vi "Laser349_RS232_Write_settings.vi"(7 "Command Status":T1, 8 "error in (no error)":errorcluster, 10 "Input value":dbl, 11 "Laser349 in":refnum<class "Laser349.lvclass">) -> (0 "error out":errorcluster, 3 "Laser349 out":refnum<class "Laser349.lvclass">)   [LabVIEW 2018, in "Laser349.lvclass"]
uses:
  Laser349.lvclass
  Ctl/_ctl_LaserCmd.ctl
  Laser349.lvclass/Laser349.ctl
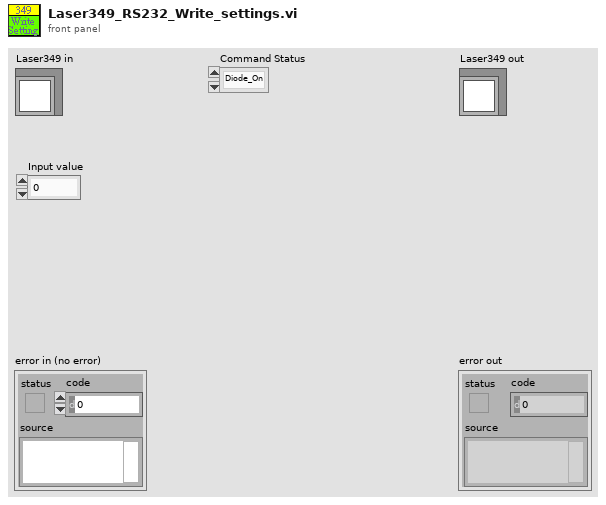
[diagram p1: front panel]
types:
  T1 = typedef "_ctl_LaserCmd.ctl" = enum8{"Diode_On", "Diode_Off", "Standby_On", "Standby_Off", "Internal_Trig", "External_Trig", "Set_Energy", "Set_Frequency", "Read_Version", "Read_STB", "Read_Diode_TEMP", "Read_SHG_TEMP", "Read_THG_TEMP", "Read_Base_Plate_TEMP", "Read_Diode_Hour", "Read_Diode_Maxc", "Read_Diode_Curr", "Read_QSW_CNTS", "Read_PENER", "Read_Freq", "Read_PCUR", "Read_Fault_Codes"}
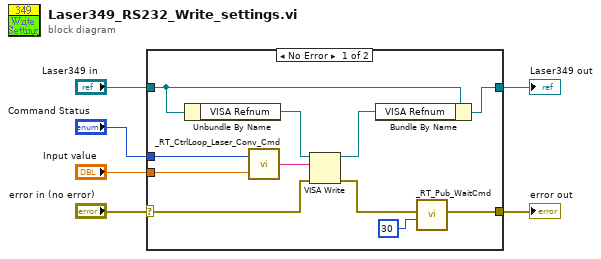
[diagram p0: block diagram]
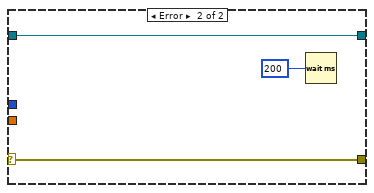
[diagram p2: hidden frame]
diagram:
  n1 = case shown="No Error" "error in (no error)" {
    selector: "error in (no error)" -> [w13 w20]
    tunnel: [w7 w20] -> w5
    tunnel: [w10 w19] -> w3
    tunnel: "Laser349 in" -> [w11 w19]
    tunnel: "Command Status" -> [w17 _]
    tunnel: "Input value" -> [w16 _]
    frame No Error {
      n2 = Unbundle By Name(w11) -> ("VISA Refnum"=w15:refnum<visa-resource-name>)
      n3 = call "_RT_CtrlLoop_Laser_Conv_Cmd.vi"("Set Value"=w16, "Command Status"=w17) -> ("Laser Command"=w14:string)
      n4 = VISA Write(VISA resource name=w15, write buffer=w14, error in (no error)=w13) -> (VISA resource name out=w12:refnum<visa-resource-name>, error out=w8:errorcluster)  [unwired: 1 out]
      n5 = Bundle By Name(cluster=w11, "VISA Refnum"=w12) -> (w10:refnum<class "Laser349.lvclass">)
      n6 = call "_RT_Pub_WaitCmd.vi"("milliseconds to wait"=u32 30, "error in (no error)"=w8) -> ("error out"=w7:errorcluster)  [unwired: 9 in]
    }
    frame Error {
      n7 = Wait (ms)(milliseconds to wait=u32 200) -> ()  [unwired: 1 out]
    }
  }
  "error out" <- w5
  "Laser349 out" <- w3
